vi "editscenario handle new scenario.vi"(6 "User Information":T4, 8 "error in (no error)":errorcluster, 10 "New Name Suggestion\n(empty - \"Username Sequence N\")":string, 11 "Connection Refnum":T5) -> (0 "error out":errorcluster, 1 "First Matching Scenario Record":T1, 2 "New Scenario Record":T1, 3 "Connection Refnum":T5, 4 "Existed?":bool)   [LabVIEW 2011]
uses:
  server/database/Scenarios/Scenario Record.ctl
  server/database/Scenarios/Conditions/Condition Record.ctl
  server/database/Scenarios/Conditions/Condition Operators.ctl
  SI.LIB/ODBC/SQL Controls/Connection Refnum.ctl
  server/database/Users/User Record.ctl
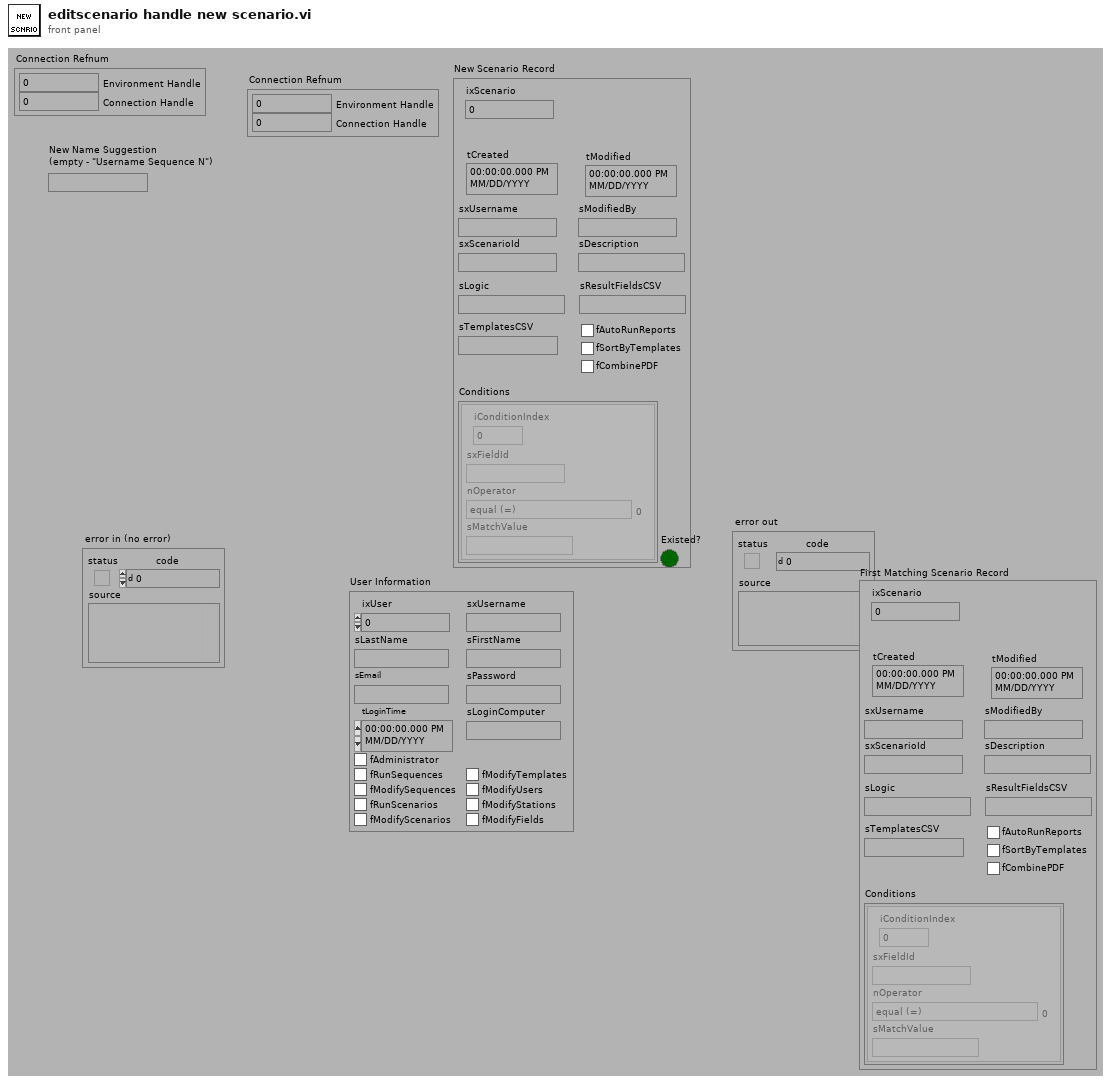
[diagram p1: front panel]
types:
  T1 = typedef "Scenario Record.ctl" = cluster{"ixScenario":i32, "tCreated":timestamp, "tModified":timestamp, "sxUsername":string, "sModifiedBy":string, "sxScenarioId":string, "sDescription":string, "sLogic":string, "sResultFieldsCSV":string, "sTemplatesCSV":string, "fAutoRunReports":bool, "fSortByTemplates":bool, "fCombinePDF":bool, "Conditions":T2[]}
  T2 = typedef "Condition Record.ctl" = cluster{"iConditionIndex":i32, "sxFieldId":string, "nOperator":T3, "sMatchValue":string}
  T3 = typedef "Condition Operators.ctl" = enum16{"equal (=)", "not equal (\\u2260)", "less than (<)", "less than or equal (\\u2264)", "greater than (>)", "greater than or equal (\\u2265)", "contains", "does not contain"}
  T4 = typedef "User Record.ctl" = cluster{"ixUser":i32, "sxUsername":string, "sLastName":string, "sFirstName":string, "sEmail":string, "sPassword":string, "tLoginTime":timestamp, "sLoginComputer":string, "fAdministrator":bool, "fRunSequences":bool, "fModifySequences":bool, "fRunScenarios":bool, "fModifyScenarios":bool, "fModifyTemplates":bool, "fModifyUsers":bool, "fModifyStations":bool, "fModifyFields":bool}
  T5 = typedef "Connection Refnum.ctl" = cluster{"Environment Handle":i32, "Connection Handle":i32}
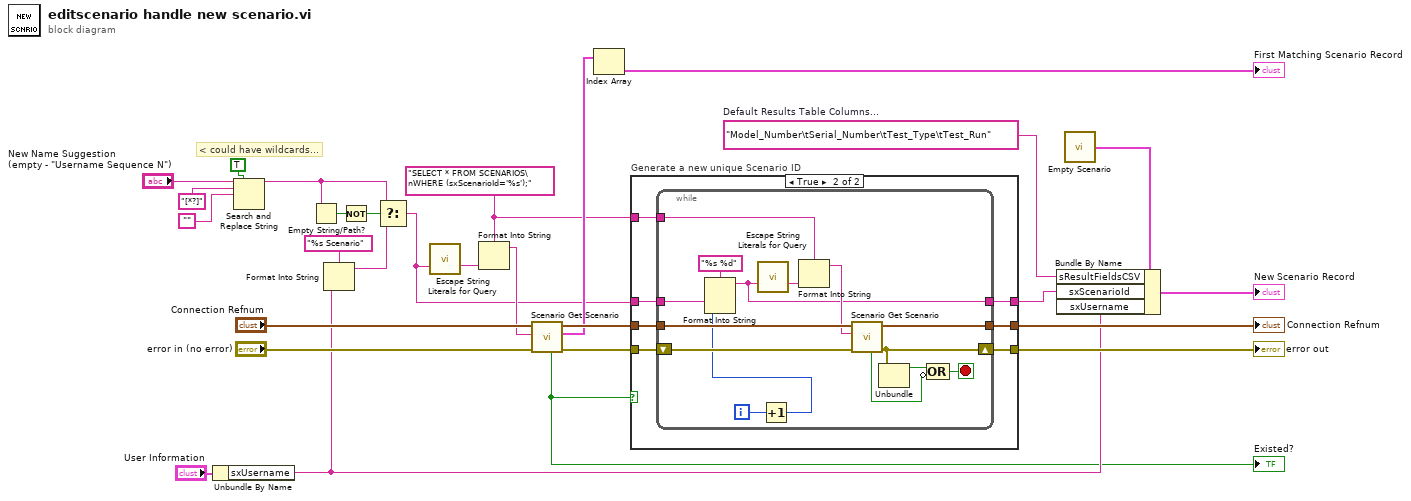
[diagram p0: block diagram]
diagram:
  w1 = "Model_Number\tSerial_Number\tTest_Type\tTest_Run"  # Default Results Table Columns...
  w7 = "SELECT * FROM SCENARIOS\nWHERE (sxScenarioId='%s');"
  # "< could have wildcards..."
  n1 = Unbundle By Name("User Information") -> ("sxUsername"=w16:string)
  n2 = Search and Replace String(replace all?=TRUE ("replace all? (F)"), input string="New Name Suggestion\n(empty - \"Username Sequence N\")", search string="[*?]", replace string="") -> (result string=w4:string)  [unwired: 1 in, 6 out]
  n3 = Empty String/Path?(string/path=w4) -> (empty?=w26:bool)
  n4 = Format Into String(format string="%s Scenario", w16) -> (resulting string=w24:string)  [unwired: 2 in, 1 out]
  n5 = Not(x=w26) -> (.not. x?=w25:bool)
  n6 = Select(t=w4, s=w25, f=w24) -> (s? t:f=w8:string)
  n7 = call "Escape String Literals for Query.vi"("String"=w8) -> ("escaped String"=w9:string)  [unwired: 1 in, 13 out]
  n8 = Format Into String(format string=w7, w9) -> (resulting string=w10:string)  [unwired: 2 in, 1 out]
  n9 = call "Scenario Get Scenario.vi"("error in (no error)"="error in (no error)", "Query"=w10, "Connection Refnum"="Connection Refnum") -> ("error out"=w19:errorcluster, "Scenarios"=w13:T1[], "Connection Refnum"=w21:T5, "Data Present?"=w15:bool)  [unwired: 5 out]
  "Existed?" <- w15
  n10 = Index Array(array=w13) -> (element=→"First Matching Scenario Record":T1)  [unwired: 1 in]
  n11 = case "Generate a new unique Scenario ID" shown="True" w15 {
    tunnel: [w31 w38] -> w23
    tunnel: [w29 w37] -> w14
    tunnel: w21 -> [w31 w36]
    tunnel: w19 -> [w30 w35]
    tunnel: [w30 w34] -> w18
    tunnel: w8 -> [w29 w32]
    tunnel: w7 -> [_ w33]
    frame False {
    }
    frame True {
      n12 = while {
        shift-right: [w47] -> w34
        shift-left: w35 -> [w46]
        tunnel: w36 -> [w49]
        tunnel: [w48] -> w38
        tunnel: [w41] -> w37
        tunnel: w33 -> [w43]
        tunnel: w32 -> [w40]
        i -> [w50]
        stop <- w51 stop-if-true
        n13 = Increment(x=w50) -> (x+1=w39:i32)
        n14 = Format Into String(format string="%s %d", w40, w39) -> (resulting string=w41:string)  [unwired: 2 in, 1 out]
        n15 = call "Escape String Literals for Query.vi"("String"=w41) -> ("escaped String"=w44:string)  [unwired: 1 in, 13 out]
        n16 = Format Into String(format string=w43, w44) -> (resulting string=w42:string)  [unwired: 2 in, 1 out]
        n17 = call "Scenario Get Scenario.vi"("error in (no error)"=w46, "Query"=w42, "Connection Refnum"=w49) -> ("error out"=w47:errorcluster, "Connection Refnum"=w48:T5, "Data Present?"=w45:bool)  [unwired: 6 out]
        n18 = Unbundle(w47) -> ("status"=w52:bool)  [unwired: 2 out]
        n19 = Compound Arithmetic op=OR(w52, invert w45) -> (w51:bool)
      }
    }
  }
  "error out" <- w18
  "Connection Refnum" <- w23
  n20 = call "Empty Scenario.vi"() -> ("Scenario Record"=w11:T1)
  n21 = Bundle By Name(cluster=w11, "sResultFieldsCSV"=w1, "sxScenarioId"=w14, "sxUsername"=w16) -> (→"New Scenario Record":T1)
